vi "动力和环境监控系统状态详情.vi"() -> ()   [LabVIEW 2016, in "环境动力监测库.lvlib"]
uses:
  <vilib>/Utility/miscctls.llb/LVRowAndColumnTypeDef.ctl
  <vilib>/ptbypt/NI_PtbyPt.lvlib
panel:
  in  "监测设备更新":bool
  in  "设备列表":i32(listbox)
  in  "add":bool
  out "设备当前时间:":timestamp format="%<%Y/%m/%d %H:%M:%S>T"
  out "当前传感器数量:":i32
  in  "设备":T1(ring)
  # "系统当前状态"
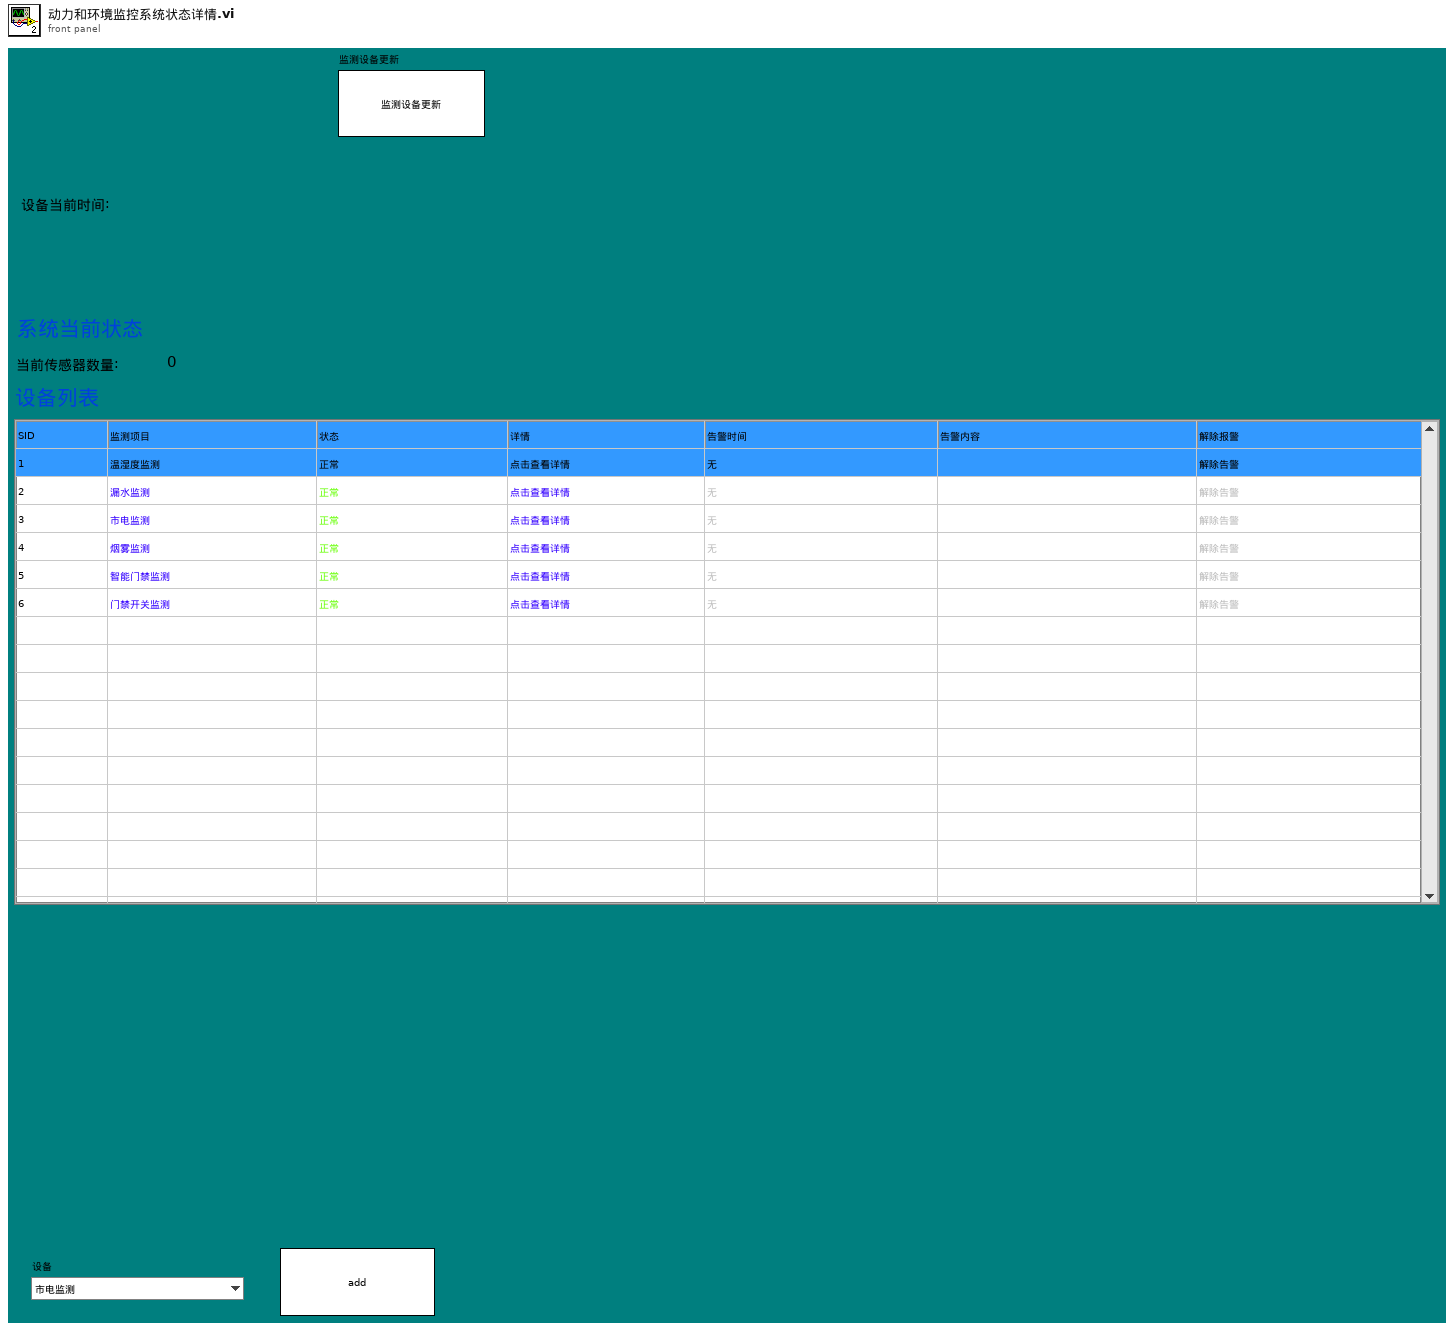
[diagram p1: front panel]
types:
  T1 = enum16{"市电监测", "UPS监测", "用水量监测", "空调监测", "烟雾监测", "温度湿度", "振动监测", "红外入侵监测", "漏水监测", "门禁开关监测", "视频监测"}
  T2 = cluster{"市电监测":bool, "用水量监测":bool, "烟雾监测":bool, "温度湿度":bool, "振动监测":bool, "红外入侵监测":bool, "漏水监测":bool, "门禁开关监测":bool, "门禁开关监测2":bool, "视频监测":bool, "UPS监测":bool, "空调监测":bool, "冰箱监测":bool, "排气扇监测":bool, "蓄电池监测":bool, "蓄电池监测2":bool, "GPS监测":bool, "北斗监测":bool, "气象监测":bool, "智能门禁监测":bool, "废液监测":bool, "废液监测2":bool, "灭火装置监测":bool}
  T3 = cluster{"漏水监测输出":cluster{"漏水监测告警":bool, "告警内容":string}, "门禁监测输出":cluster{"门禁监测告警":bool, "告警内容":string}, "门禁监测输出2":cluster{"门禁监测告警":bool, "告警内容":string}, "温湿度监测输出":cluster{"温湿度监测告警":bool, "告警内容":string}, "烟雾监测输出":cluster{"烟雾监测告警":bool, "告警内容":string}, "空调监测输出":cluster{"空调监测告警":bool, "告警内容":string}, "自动重合闸输出":cluster{"自动重合闸告警":bool, "告警内容":string}, "红外入侵输出":cluster{"红外入侵告警":bool, "告警内容":string}, "振动输出":cluster{"振动告警":bool, "告警内容":string}, "UPS输出":cluster{"UPS告警":bool, "告警内容":string}, "蓄电池输出":cluster{"蓄电池告警":bool, "告警内容":string}, "蓄电池输出2":cluster{"蓄电池告警":bool, "告警内容":string}, "GPS输出":cluster{"定位告警":bool, "告警内容":string}, "北斗输出":cluster{"定位告警":bool, "告警内容":string}, "气象输出":cluster{"气象告警":bool, "告警内容":string}, "废液输出":cluster{"废液告警":bool, "告警内容":string}, "废液输出2":cluster{"废液告警":bool, "告警内容":string}, "灭火装置输出":cluster{"灭火装置告警":bool, "告警内容":string}}
  T4 = cluster{"温湿度":cluster{"状态":bool, "温度:":sgl, "湿度:":sgl, "详情  ":bool}, "空调":cluster{"状态":bool, "机柜温度:":sgl, "压缩机:":enum16{"停止", "运行"}, "电加热:":enum16{"停止", "运行"}, "详情  ":bool}, "排气扇":cluster{"排气扇":bool, "详情  ":bool}, "冰箱":cluster{"冰箱":bool, "详情  ":bool}}
  T5 = cluster{"市电":cluster{"状态":bool, "电压:":u16, "电流：":dbl, "详情  ":bool}, "UPS":cluster{"状态":bool, "输入电压:":sgl, "输出电压:":sgl, "电池电量:":u8, "电量":u16, "详情  ":bool}, "蓄电池12V":cluster{"状态":bool, "电压:":sgl, "电流:":sgl, "电池电量:":u8, "电量":u16, "详情  ":bool, "充电":bool, "负载":bool}, "蓄电池24V":cluster{"状态":bool, "电压:":sgl, "电流:":sgl, "电池电量:":u8, "电量":u16, "详情  ":bool, "充电":bool, "负载":bool}}
  T6 = cluster{"传感器":cluster{"红外监测":cluster{"红外监测":bool, "红外入侵监测":bool}, "振动监测":cluster{"振动监测":bool, "振动监测 2":bool}, "烟雾监测":cluster{"烟雾监测":bool, "烟雾监测 2":bool}, "门禁监测":cluster{"门禁监测":bool, "门禁开关监测":bool}, "门禁2监测":cluster{"门禁监测2":bool, "门禁开关监测2":bool}, "水浸监测":cluster{"水浸监测":bool, "漏水详情":bool}, "废液监测":cluster{"废液监测":bool, "废液详情":bool}, "废液监测2":cluster{"废液监测2":bool, "废液2详情":bool}, "灭火装置":cluster{"灭火装置":bool, "灭火装置详情":bool}}, "气象仪":cluster{"气温: ":sgl, "气压: ":sgl, "风速:":sgl, "风向:":sgl, "气象仪经度: ":sgl, "气象仪纬度: ":sgl, "详情  ":bool}}
  T7 = cluster{"AD0":dbl, "AD1":dbl, "AD2":dbl, "AD3":dbl, "AD4":dbl, "AD5":dbl, "AD6":dbl, "AD7":dbl}
  T8 = cluster{"X0":dbl, "X1":dbl, "Y0":dbl, "Y1":dbl}[]
  T9 = enum32{"Invalid", "Standard", "Closed", "Hidden", "Minimized", "Maximized"}
  T10 = typedef "LVRowAndColumnTypeDef.ctl" = cluster{"Row":i32, "Column":i32}
  T11 = typedef "LVPoint32TypeDef.ctl" = cluster{"Horizontal":i32, "Vertical":i32}
  T12 = enum32{"Bad", "Idle", "Run top level", "Running"}
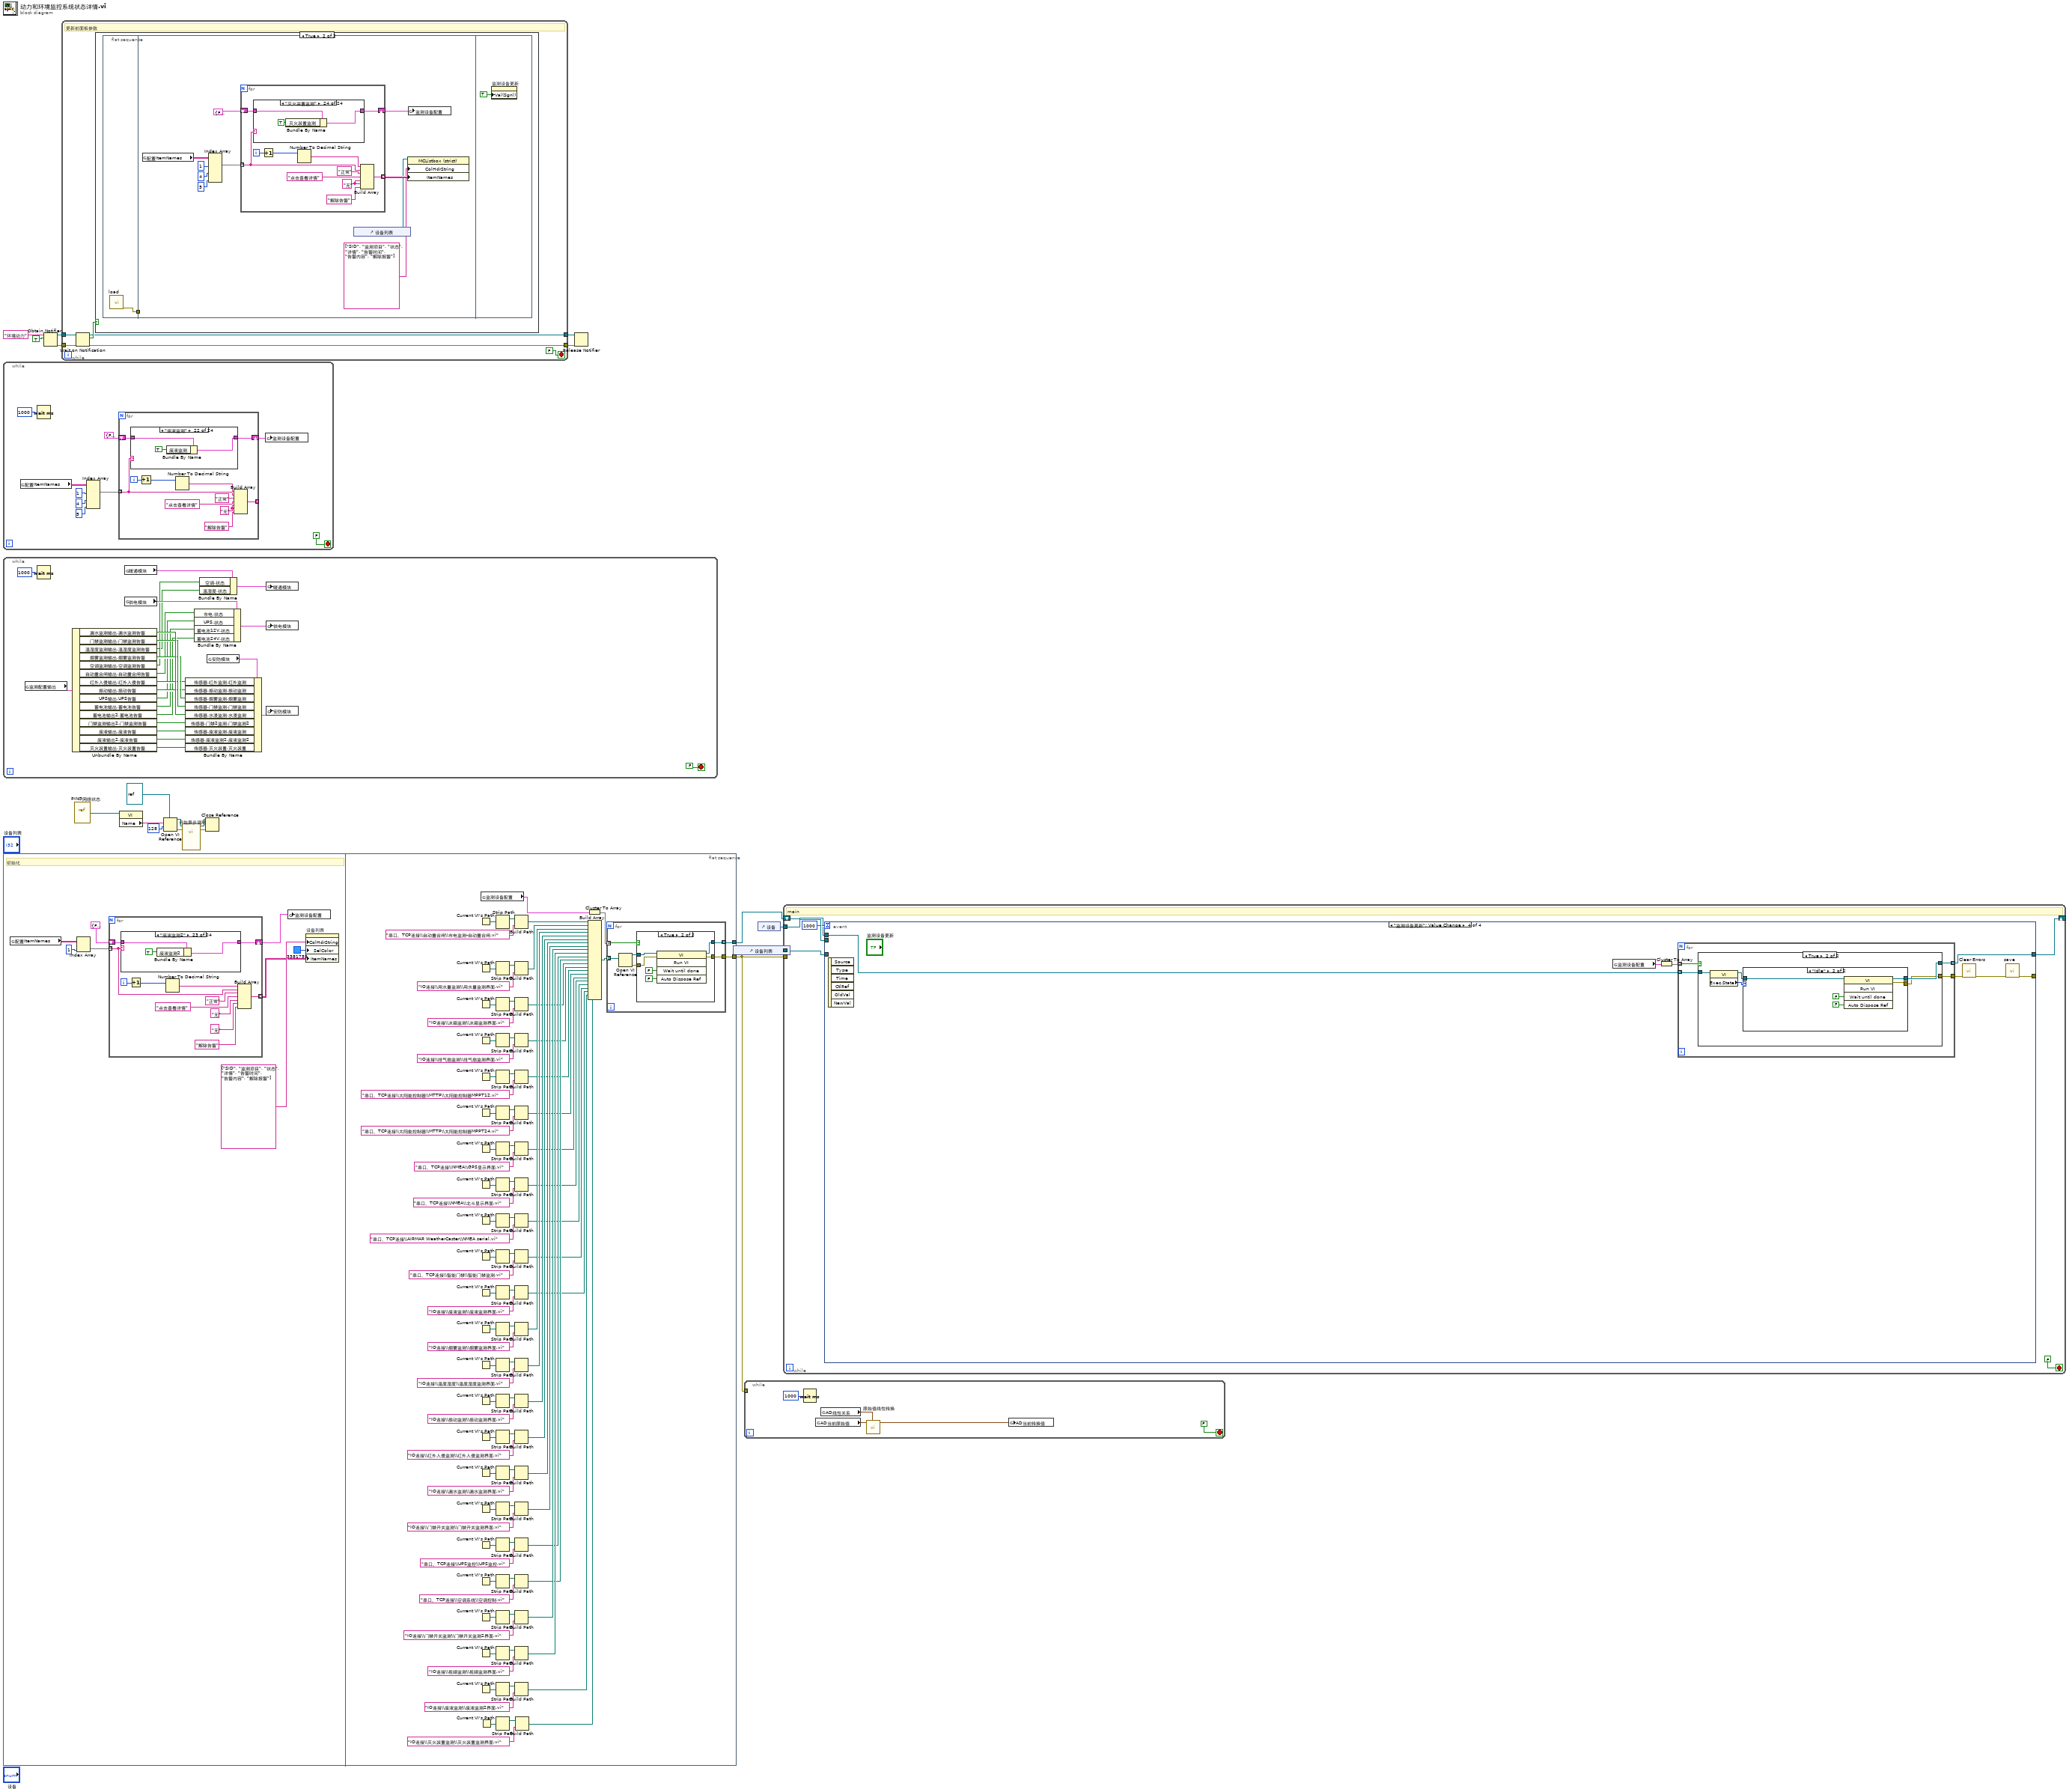
[diagram p0: block diagram]
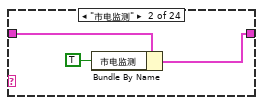
[diagram p3: hidden frame]
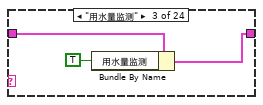
[diagram p4: hidden frame]
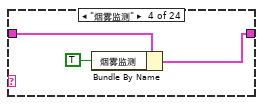
[diagram p5: hidden frame]
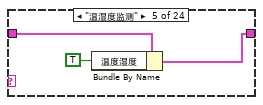
[diagram p6: hidden frame]
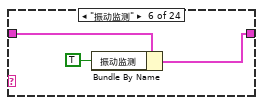
[diagram p7: hidden frame]
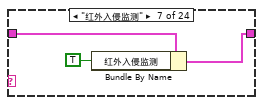
[diagram p8: hidden frame]
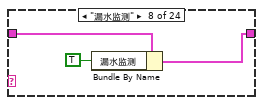
[diagram p9: hidden frame]
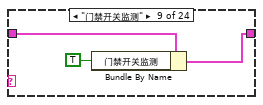
[diagram p10: hidden frame]
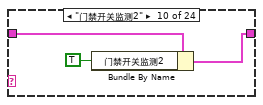
[diagram p11: hidden frame]
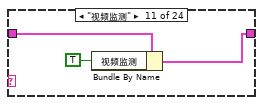
[diagram p12: hidden frame]
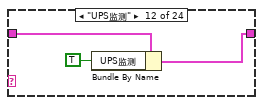
[diagram p13: hidden frame]
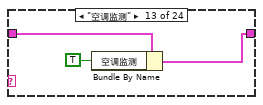
[diagram p14: hidden frame]
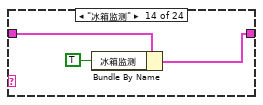
[diagram p15: hidden frame]
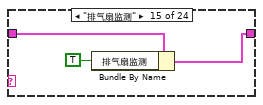
[diagram p16: hidden frame]
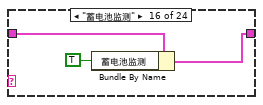
[diagram p17: hidden frame]
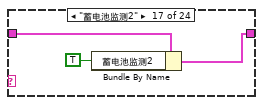
[diagram p18: hidden frame]
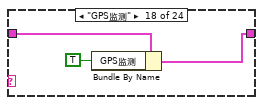
[diagram p19: hidden frame]
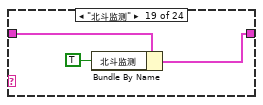
[diagram p20: hidden frame]
diagram:
  n1 = while {
    stop <- FALSE stop-if-true
    n2 = global read "断电保存全局变量.vi" "配置ItemNames"() -> (w22:string[][])
    n3 = Wait (ms)(milliseconds to wait=u32 1000 ("等待时间（毫秒）")) -> ()  [unwired: 1 out]
    n4 = Index Array(array=w22, index (col) #1=1 ("禁用的索引 (列)"), index (col) #2=4 ("索引 (列)"), index (col) #3=5 ("索引 (列)")) -> (element #1=w20:string[])  [unwired: 3 in, 2 out]
    n5 = for {
      tunnel: w20 -> [w29] mode=indexing
      tunnel: [w33] -> _ mode=indexing
      shift-right: [w28] -> w23
      shift-left: T2 {"市电监测"=FALSE, "用水量监测"=FALSE, "烟雾监测"=FALSE, "温度湿度"=FALSE, "振动监测"=FALSE, "红外入侵监测"=FALSE, "漏水监测"=FALSE, "门禁开关监测"=FALSE, "门禁开关监测2"=FALSE, "视频监测"=FALSE, "UPS监测"=FALSE, "空调监测"=FALSE, "冰箱监测"=FALSE, "排气扇监测"=FALSE, "蓄电池监测"=FALSE, "蓄电池监测2"=FALSE, "GPS监测"=FALSE, "北斗监测"=FALSE, "气象监测"=FALSE, "智能门禁监测"=FALSE, "废液监测"=FALSE, "废液监测2"=FALSE, "灭火装置监测"=FALSE} ("监测设备配置") -> [w30]
      i -> [w38]
      w31 = "无" ("元素")
      n6 = case shown="\"废液监测\"" w29 {
        tunnel: w30 -> [w39 w42 w44 w47 w50 w53 w56 w59 w62 w65 w68 w71 w74 w77 w80 w83 w86 w89 w92 w95 w98 w101 w104 w107]
        tunnel: [w39 w40 w43 w46 w49 w52 w55 w58 w61 w64 w67 w70 w73 w76 w79 w82 w85 w88 w91 w94 w97 w100 w103 w106] -> w28
        frame "假", Default {
        }
        frame "市电监测" {
          n7 = Bundle By Name(cluster=w42, "市电监测"=TRUE) -> (w40:T2)
        }
        frame "用水量监测" {
          n8 = Bundle By Name(cluster=w44, "用水量监测"=TRUE ("市电监测")) -> (w43:T2)
        }
        frame "烟雾监测" {
          n9 = Bundle By Name(cluster=w47, "烟雾监测"=TRUE ("市电监测")) -> (w46:T2)
        }
        frame "温湿度监测" {
          n10 = Bundle By Name(cluster=w50, "温度湿度"=TRUE ("市电监测")) -> (w49:T2)
        }
        frame "振动监测" {
          n11 = Bundle By Name(cluster=w53, "振动监测"=TRUE ("市电监测")) -> (w52:T2)
        }
        frame "红外入侵监测" {
          n12 = Bundle By Name(cluster=w56, "红外入侵监测"=TRUE ("市电监测")) -> (w55:T2)
        }
        frame "漏水监测" {
          n13 = Bundle By Name(cluster=w59, "漏水监测"=TRUE ("市电监测")) -> (w58:T2)
        }
        frame "门禁开关监测" {
          n14 = Bundle By Name(cluster=w62, "门禁开关监测"=TRUE ("市电监测")) -> (w61:T2)
        }
        frame "门禁开关监测2" {
          n15 = Bundle By Name(cluster=w65, "门禁开关监测2"=TRUE ("市电监测")) -> (w64:T2)
        }
        frame "视频监测" {
          n16 = Bundle By Name(cluster=w68, "视频监测"=TRUE ("市电监测")) -> (w67:T2)
        }
        frame "UPS监测" {
          n17 = Bundle By Name(cluster=w71, "UPS监测"=TRUE ("市电监测")) -> (w70:T2)
        }
        frame "空调监测" {
          n18 = Bundle By Name(cluster=w74, "空调监测"=TRUE ("市电监测")) -> (w73:T2)
        }
        frame "冰箱监测" {
          n19 = Bundle By Name(cluster=w77, "冰箱监测"=TRUE ("市电监测")) -> (w76:T2)
        }
        frame "排气扇监测" {
          n20 = Bundle By Name(cluster=w80, "排气扇监测"=TRUE ("市电监测")) -> (w79:T2)
        }
        frame "蓄电池监测" {
          n21 = Bundle By Name(cluster=w83, "蓄电池监测"=TRUE ("市电监测")) -> (w82:T2)
        }
        frame "蓄电池监测2" {
          n22 = Bundle By Name(cluster=w86, "蓄电池监测2"=TRUE ("市电监测")) -> (w85:T2)
        }
        frame "GPS监测" {
          n23 = Bundle By Name(cluster=w89, "GPS监测"=TRUE ("市电监测")) -> (w88:T2)
        }
        frame "北斗监测" {
          n24 = Bundle By Name(cluster=w92, "北斗监测"=TRUE ("市电监测")) -> (w91:T2)
        }
        frame "气象监测" {
          n25 = Bundle By Name(cluster=w95, "气象监测"=TRUE ("市电监测")) -> (w94:T2)
        }
        frame "智能门禁监测" {
          n26 = Bundle By Name(cluster=w98, "智能门禁监测"=TRUE ("市电监测")) -> (w97:T2)
        }
        frame "废液监测" {
          n27 = Bundle By Name(cluster=w101, "废液监测"=TRUE ("市电监测")) -> (w100:T2)
        }
        frame "废液监测2" {
          n28 = Bundle By Name(cluster=w104, "废液监测2"=TRUE ("市电监测")) -> (w103:T2)
        }
        frame "灭火装置监测" {
          n29 = Bundle By Name(cluster=w107, "灭火装置监测"=TRUE ("市电监测")) -> (w106:T2)
        }
      }
      n30 = Increment(x=w38) -> (x+1=w37:i32)
      n31 = Number To Decimal String(number=w37) -> (decimal integer string=w36:string)  [unwired: 1 in]
      n32 = Build Array(w36, w29, "正常" ("元素"), "点击查看详情" ("元素"), w31, w31, "解除告警" ("元素")) -> (w33:string[])
    }
    n33 = global write "断电保存全局变量.vi" "监测设备配置"(w23) -> ()
  }
  n34 = while {
    stop <- FALSE stop-if-true
    n35 = global read "内部交互全局变量.vi" "监测配置输出"() -> (w113:T3)
    n36 = Wait (ms)(milliseconds to wait=u32 1000 ("等待时间（毫秒）")) -> ()  [unwired: 1 out]
    n37 = Unbundle By Name(w113) -> ("漏水监测输出.漏水监测告警"=w128:bool, "门禁监测输出.门禁监测告警"=w127:bool, "温湿度监测输出.温湿度监测告警"=w115:bool, "烟雾监测输出.烟雾监测告警"=w126:bool, "空调监测输出.空调监测告警"=w116:bool, "自动重合闸输出.自动重合闸告警"=w121:bool, "红外入侵输出.红外入侵告警"=w125:bool, "振动输出.振动告警"=w124:bool, "UPS输出.UPS告警"=w120:bool, "蓄电池输出.蓄电池告警"=w119:bool, "蓄电池输出2.蓄电池告警"=w114:bool, "门禁监测输出2.门禁监测告警"=w112:bool, "废液输出.废液告警"=w111:bool, "废液输出2.废液告警"=w110:bool, "灭火装置输出.灭火装置告警"=w109:bool)
    n38 = global read "内部交互全局变量.vi" "暖通模块"() -> (w118:T4)
    n39 = global read "内部交互全局变量.vi" "供电模块"() -> (w122:T5)
    n40 = Bundle By Name(cluster=w122, "市电.状态"=w121, "UPS.状态"=w120, "蓄电池12V.状态"=w119, "蓄电池24V.状态"=w114) -> (w123:T5)
    n41 = Bundle By Name(cluster=w118, "空调.状态"=w116, "温湿度.状态"=w115) -> (w117:T4)
    n42 = global read "内部交互全局变量.vi" "安防模块"() -> (w130:T6)
    n43 = Bundle By Name(cluster=w130, "传感器.红外监测.红外监测"=w125, "传感器.振动监测.振动监测"=w124, "传感器.烟雾监测.烟雾监测"=w126, "传感器.门禁监测.门禁监测"=w127, "传感器.水浸监测.水浸监测"=w128, "传感器.门禁2监测.门禁监测2"=w112, "传感器.废液监测.废液监测"=w111, "传感器.废液监测2.废液监测2"=w110, "传感器.灭火装置.灭火装置"=w109) -> (w129:T6)
    n44 = global write "内部交互全局变量.vi" "暖通模块"(w117) -> ()
    n45 = global write "内部交互全局变量.vi" "供电模块"(w123) -> ()
    n46 = global write "内部交互全局变量.vi" "安防模块"(w129) -> ()
  }
  n47 = flat-sequence {
    tunnel: [w317] -> w12
    tunnel: [w227] -> w1
    frame #0 {
      # "初始化"
      n48 = global read "断电保存全局变量.vi" "配置ItemNames"() -> (w138:string[][])
      n49 = Index Array(array=w138, index (col)=1 ("禁用的索引 (列)")) -> (element=w136:string[])  [unwired: 1 in]
      n50 = for {
        tunnel: w136 -> [w143] mode=indexing
        tunnel: [w147] -> w135 mode=indexing
        shift-right: [w141] -> w133
        shift-left: T2 {"市电监测"=FALSE, "用水量监测"=FALSE, "烟雾监测"=FALSE, "温度湿度"=FALSE, "振动监测"=FALSE, "红外入侵监测"=FALSE, "漏水监测"=FALSE, "门禁开关监测"=FALSE, "门禁开关监测2"=FALSE, "视频监测"=FALSE, "UPS监测"=FALSE, "空调监测"=FALSE, "冰箱监测"=FALSE, "排气扇监测"=FALSE, "蓄电池监测"=FALSE, "蓄电池监测2"=FALSE, "GPS监测"=FALSE, "北斗监测"=FALSE, "气象监测"=FALSE, "智能门禁监测"=FALSE, "废液监测"=FALSE, "废液监测2"=FALSE, "灭火装置监测"=FALSE} ("监测设备配置") -> [w142]
        i -> [w152]
        n51 = case shown="\"废液监测2\"" w143 {
          tunnel: w142 -> [w153 w156 w158 w161 w164 w167 w170 w173 w176 w179 w182 w185 w188 w191 w194 w197 w200 w203 w206 w209 w212 w215 w218 w221]
          tunnel: [w153 w154 w157 w160 w163 w166 w169 w172 w175 w178 w181 w184 w187 w190 w193 w196 w199 w202 w205 w208 w211 w214 w217 w220] -> w141
          frame "假", Default {
          }
          frame "市电监测" {
            n52 = Bundle By Name(cluster=w156, "市电监测"=TRUE) -> (w154:T2)
          }
          frame "用水量监测" {
            n53 = Bundle By Name(cluster=w158, "用水量监测"=TRUE ("市电监测")) -> (w157:T2)
          }
          frame "烟雾监测" {
            n54 = Bundle By Name(cluster=w161, "烟雾监测"=TRUE ("市电监测")) -> (w160:T2)
          }
          frame "温湿度监测" {
            n55 = Bundle By Name(cluster=w164, "温度湿度"=TRUE ("市电监测")) -> (w163:T2)
          }
          frame "振动监测" {
            n56 = Bundle By Name(cluster=w167, "振动监测"=TRUE ("市电监测")) -> (w166:T2)
          }
          frame "红外入侵监测" {
            n57 = Bundle By Name(cluster=w170, "红外入侵监测"=TRUE ("市电监测")) -> (w169:T2)
          }
          frame "漏水监测" {
            n58 = Bundle By Name(cluster=w173, "漏水监测"=TRUE ("市电监测")) -> (w172:T2)
          }
          frame "门禁开关监测" {
            n59 = Bundle By Name(cluster=w176, "门禁开关监测"=TRUE ("市电监测")) -> (w175:T2)
          }
          frame "门禁开关监测2" {
            n60 = Bundle By Name(cluster=w179, "门禁开关监测2"=TRUE ("市电监测")) -> (w178:T2)
          }
          frame "视频监测" {
            n61 = Bundle By Name(cluster=w182, "视频监测"=TRUE ("市电监测")) -> (w181:T2)
          }
          frame "UPS监测" {
            n62 = Bundle By Name(cluster=w185, "UPS监测"=TRUE ("市电监测")) -> (w184:T2)
          }
          frame "空调监测" {
            n63 = Bundle By Name(cluster=w188, "空调监测"=TRUE ("市电监测")) -> (w187:T2)
          }
          frame "冰箱监测" {
            n64 = Bundle By Name(cluster=w191, "冰箱监测"=TRUE ("市电监测")) -> (w190:T2)
          }
          frame "排气扇监测" {
            n65 = Bundle By Name(cluster=w194, "排气扇监测"=TRUE ("市电监测")) -> (w193:T2)
          }
          frame "蓄电池监测" {
            n66 = Bundle By Name(cluster=w197, "蓄电池监测"=TRUE ("市电监测")) -> (w196:T2)
          }
          frame "蓄电池监测2" {
            n67 = Bundle By Name(cluster=w200, "蓄电池监测2"=TRUE ("市电监测")) -> (w199:T2)
          }
          frame "GPS监测" {
            n68 = Bundle By Name(cluster=w203, "GPS监测"=TRUE ("市电监测")) -> (w202:T2)
          }
          frame "北斗监测" {
            n69 = Bundle By Name(cluster=w206, "北斗监测"=TRUE ("市电监测")) -> (w205:T2)
          }
          frame "气象监测" {
            n70 = Bundle By Name(cluster=w209, "气象监测"=TRUE ("市电监测")) -> (w208:T2)
          }
          frame "智能门禁监测" {
            n71 = Bundle By Name(cluster=w212, "智能门禁监测"=TRUE ("市电监测")) -> (w211:T2)
          }
          frame "废液监测" {
            n72 = Bundle By Name(cluster=w215, "废液监测"=TRUE ("市电监测")) -> (w214:T2)
          }
          frame "废液监测2" {
            n73 = Bundle By Name(cluster=w218, "废液监测2"=TRUE ("市电监测")) -> (w217:T2)
          }
          frame "灭火装置监测" {
            n74 = Bundle By Name(cluster=w221, "灭火装置监测"=TRUE ("市电监测")) -> (w220:T2)
          }
        }
        n75 = Increment(x=w152) -> (x+1=w151:i32)
        n76 = Number To Decimal String(number=w151) -> (decimal integer string=w150:string)  [unwired: 1 in]
        n77 = Build Array(w150, w143, "正常" ("元素"), "点击查看详情" ("元素"), "无" ("元素"), "无" ("元素"), "解除告警" ("元素")) -> (w147:string[])
      }
      n78 = global write "断电保存全局变量.vi" "监测设备配置"(w133) -> ()
      n79 = property on="设备列表" class="MCListbox (strict)"("ColHdrString"=string[] ["SID", "监测项目", "状态", "详情", "告警时间", "告警内容", "解除报警"] ("列首字符串[]"), "SelColor"=u32 3381759, "ItemNames"=w135) -> ()  [unwired: 2 in, 2 out]
    }
    frame #1 {
      n80 = Current VI's Path() -> (path=w315:path)
      n81 = Current VI's Path() -> (path=w309:path)
      n82 = Current VI's Path() -> (path=w264:path)
      n83 = Current VI's Path() -> (path=w265:path)
      n84 = Current VI's Path() -> (path=w259:path)
      n85 = Current VI's Path() -> (path=w254:path)
      n86 = Current VI's Path() -> (path=w251:path)
      n87 = Current VI's Path() -> (path=w245:path)
      n88 = Current VI's Path() -> (path=w243:path)
      n89 = Current VI's Path() -> (path=w237:path)
      n90 = Current VI's Path() -> (path=w235:path)
      n91 = Current VI's Path() -> (path=w307:path)
      n92 = Current VI's Path() -> (path=w301:path)
      n93 = Current VI's Path() -> (path=w299:path)
      n94 = Current VI's Path() -> (path=w293:path)
      n95 = Current VI's Path() -> (path=w289:path)
      n96 = Current VI's Path() -> (path=w287:path)
      n97 = Current VI's Path() -> (path=w275:path)
      n98 = Current VI's Path() -> (path=w269:path)
      n99 = Current VI's Path() -> (path=w281:path)
      n100 = Current VI's Path() -> (path=w279:path)
      n101 = Current VI's Path() -> (path=w230:path)
      n102 = Current VI's Path() -> (path=w226:path)
      n103 = global read "断电保存全局变量.vi" "监测设备配置"() -> (w316:T2)
      n104 = Strip Path(path=w315) -> (stripped path=w314:path)  [unwired: 1 out]
      n105 = Strip Path(path=w309) -> (stripped path=w310:path)  [unwired: 1 out]
      n106 = Strip Path(path=w264) -> (stripped path=w263:path)  [unwired: 1 out]
      n107 = Strip Path(path=w265) -> (stripped path=w266:path)  [unwired: 1 out]
      n108 = Strip Path(path=w259) -> (stripped path=w258:path)  [unwired: 1 out]
      n109 = Strip Path(path=w254) -> (stripped path=w255:path)  [unwired: 1 out]
      n110 = Strip Path(path=w251) -> (stripped path=w250:path)  [unwired: 1 out]
      n111 = Strip Path(path=w245) -> (stripped path=w246:path)  [unwired: 1 out]
      n112 = Strip Path(path=w243) -> (stripped path=w242:path)  [unwired: 1 out]
      n113 = Strip Path(path=w237) -> (stripped path=w238:path)  [unwired: 1 out]
      n114 = Strip Path(path=w235) -> (stripped path=w234:path)  [unwired: 1 out]
      n115 = Strip Path(path=w307) -> (stripped path=w306:path)  [unwired: 1 out]
      n116 = Strip Path(path=w301) -> (stripped path=w302:path)  [unwired: 1 out]
      n117 = Strip Path(path=w299) -> (stripped path=w298:path)  [unwired: 1 out]
      n118 = Strip Path(path=w293) -> (stripped path=w294:path)  [unwired: 1 out]
      n119 = Strip Path(path=w289) -> (stripped path=w290:path)  [unwired: 1 out]
      n120 = Strip Path(path=w287) -> (stripped path=w286:path)  [unwired: 1 out]
      n121 = Strip Path(path=w275) -> (stripped path=w274:path)  [unwired: 1 out]
      n122 = Strip Path(path=w269) -> (stripped path=w270:path)  [unwired: 1 out]
      n123 = Strip Path(path=w281) -> (stripped path=w282:path)  [unwired: 1 out]
      n124 = Strip Path(path=w279) -> (stripped path=w278:path)  [unwired: 1 out]
      n125 = Strip Path(path=w230) -> (stripped path=w231:path)  [unwired: 1 out]
      n126 = Strip Path(path=w226) -> (stripped path=w225:path)  [unwired: 1 out]
      n127 = Build Path(base path=w314, name or relative path="串口、TCP连接\\自动重合闸\\市电监测-自动重合闸.vi" ("名称或相对路径")) -> (appended path=w312:path)
      n128 = Build Path(base path=w310, name or relative path="IO连接\\用水量监测\\用水量监测界面.vi" ("名称或相对路径")) -> (appended path=w308:path)
      n129 = Build Path(base path=w263, name or relative path="IO连接\\冰箱监测\\冰箱监测界面.vi" ("名称或相对路径")) -> (appended path=w261:path)
      n130 = Build Path(base path=w266, name or relative path="IO连接\\排气扇监测\\排气扇监测界面.vi" ("名称或相对路径")) -> (appended path=w260:path)
      n131 = Build Path(base path=w258, name or relative path="串口、TCP连接\\太阳能控制器\\MTTP\\太阳能控制器MPPT12.vi" ("名称或相对路径")) -> (appended path=w253:path)
      n132 = Build Path(base path=w255, name or relative path="串口、TCP连接\\太阳能控制器\\MTTP\\太阳能控制器MPPT24.vi" ("名称或相对路径")) -> (appended path=w252:path)
      n133 = Build Path(base path=w250, name or relative path="串口、TCP连接\\NMEA\\GPS显示界面.vi" ("名称或相对路径")) -> (appended path=w248:path)
      n134 = Build Path(base path=w246, name or relative path="串口、TCP连接\\NMEA\\北斗显示界面.vi" ("名称或相对路径")) -> (appended path=w244:path)
      n135 = Build Path(base path=w242, name or relative path="串口、TCP连接\\AIRMAR WeatherCaster\\NMEA serial.vi" ("名称或相对路径")) -> (appended path=w240:path)
      n136 = Build Path(base path=w238, name or relative path="串口、TCP连接\\智能门禁\\智能门禁监测.vi" ("名称或相对路径")) -> (appended path=w236:path)
      n137 = Build Path(base path=w234, name or relative path="IO连接\\废液监测\\废液监测界面.vi" ("名称或相对路径")) -> (appended path=w229:path)
      n138 = Build Path(base path=w306, name or relative path="IO连接\\烟雾监测\\烟雾监测界面.vi" ("名称或相对路径")) -> (appended path=w304:path)
      n139 = Build Path(base path=w302, name or relative path="IO连接\\温度湿度\\温度湿度监测界面.vi" ("名称或相对路径")) -> (appended path=w300:path)
      n140 = Build Path(base path=w298, name or relative path="IO连接\\振动监测\\振动监测界面.vi" ("名称或相对路径")) -> (appended path=w296:path)
      n141 = Build Path(base path=w294, name or relative path="IO连接\\红外入侵监测\\红外入侵监测界面.vi" ("名称或相对路径")) -> (appended path=w292:path)
      n142 = Build Path(base path=w290, name or relative path="IO连接\\漏水监测\\漏水监测界面.vi" ("名称或相对路径")) -> (appended path=w288:path)
      n143 = Build Path(base path=w286, name or relative path="IO连接\\门禁开关监测\\门禁开关监测界面.vi" ("名称或相对路径")) -> (appended path=w284:path)
      n144 = Build Path(base path=w274, name or relative path="串口、TCP连接\\UPS监控\\UPS监控.vi" ("名称或相对路径")) -> (appended path=w272:path)
      n145 = Build Path(base path=w270, name or relative path="串口、TCP连接\\空调系统\\空调控制.vi" ("名称或相对路径")) -> (appended path=w268:path)
      n146 = Build Path(base path=w282, name or relative path="IO连接\\门禁开关监测\\门禁开关监测2界面.vi" ("名称或相对路径")) -> (appended path=w280:path)
      n147 = Build Path(base path=w278, name or relative path="IO连接\\视频监测\\视频监测界面.vi" ("名称或相对路径")) -> (appended path=w276:path)
      n148 = Build Path(base path=w231, name or relative path="IO连接\\废液监测\\废液监测2界面.vi" ("名称或相对路径")) -> (appended path=w228:path)
      n149 = Build Path(base path=w225, name or relative path="IO连接\\灭火装置监测\\灭火装置监测界面.vi" ("名称或相对路径")) -> (appended path=w223:path)
      n150 = Cluster To Array(cluster=w316) -> (array=w319:bool[])
      n151 = Build Array(w312, w308, w304, w300, w296, w292, w288, w284, w280, w276, w272, w268, w261, w260, w253, w252, w248, w244, w240, w236, w229, w228, w223) -> (w318:path[])
      n152 = for {
        tunnel: w318 -> [w322] mode=indexing
        tunnel: [w321] -> w317 mode=indexing
        tunnel: w319 -> [w325] mode=indexing
        tunnel: [w320] -> w227
        n153 = Open VI Reference(vi path=w322) -> (vi reference=w324:refnum<vi>, error out=w323:errorcluster)  [unwired: 5 in]
        n154 = case shown="True" w325 {
          tunnel: w324 -> [w326 w330]
          tunnel: [w326 w329] -> w321
          tunnel: [_ w328] -> w320
          tunnel: w323 -> [_ w327]
          frame False {
          }
          frame True {
            n155 = invoke class="VI" method="Run VI"(reference=w330, error in=w327, "Wait until done"=FALSE ("结束前等待"), "Auto Dispose Ref"=FALSE ("自动销毁引用")) -> (reference out=w329:refnum<vi>, error out=w328:errorcluster)  [unwired: 1 in, 3 out]
          }
        }
      }
    }
  }
  n156 = Obtain Notifier(name (unnamed)="环境动力" ("名称（未命名）"), notification data type=TRUE) -> (notifier out=w3:refnum<notifier>, error out=w2:errorcluster)  [unwired: 2 in, 1 out]
  n157 = while {
    tunnel: w3 -> [w338]
    tunnel: w2 -> [w337]
    tunnel: [w334] -> w14
    tunnel: [w333] -> w13
    stop <- FALSE stop-if-true
    # "更新前面板参数"
    n158 = Wait on Notification(notifier=w338, error in (no error)=w337) -> (notifier out=w334:refnum<notifier>, notification=w336:bool, error out=w333:errorcluster)  [unwired: 2 in, 1 out]
    n159 = case shown="True" w336 {
      frame False {
      }
      frame True {
        n160 = flat-sequence {
          tunnel: [w340] -> w339
          tunnel: w339 -> [_]
          frame #0 {
            n161 = call "load.vi"() -> ("error out"=w340:errorcluster)  [unwired: 11 in]
          }
          frame #1 {
            n162 = global read "断电保存全局变量.vi" "配置ItemNames"() -> (w345:string[][])
            n163 = Index Array(array=w345, index (col) #1=1 ("禁用的索引 (列)"), index (col) #2=4 ("索引 (列)"), index (col) #3=5 ("索引 (列)")) -> (element #1=w347:string[])  [unwired: 3 in, 2 out]
            n164 = for {
              tunnel: w347 -> [w352] mode=indexing
              tunnel: [w356] -> w350 mode=indexing
              shift-right: [w351] -> w342
              shift-left: T2 {"市电监测"=FALSE, "用水量监测"=FALSE, "烟雾监测"=FALSE, "温度湿度"=FALSE, "振动监测"=FALSE, "红外入侵监测"=FALSE, "漏水监测"=FALSE, "门禁开关监测"=FALSE, "门禁开关监测2"=FALSE, "视频监测"=FALSE, "UPS监测"=FALSE, "空调监测"=FALSE, "冰箱监测"=FALSE, "排气扇监测"=FALSE, "蓄电池监测"=FALSE, "蓄电池监测2"=FALSE, "GPS监测"=FALSE, "北斗监测"=FALSE, "气象监测"=FALSE, "智能门禁监测"=FALSE, "废液监测"=FALSE, "废液监测2"=FALSE, "灭火装置监测"=FALSE} ("监测设备配置") -> [w353]
              i -> [w361]
              w354 = "无" ("元素")
              n165 = case shown="\"灭火装置监测\"" w352 {
                tunnel: w353 -> [w362 w365 w367 w370 w373 w376 w379 w382 w385 w388 w391 w394 w397 w400 w403 w406 w409 w412 w415 w418 w421 w424 w427 w430]
                tunnel: [w362 w363 w366 w369 w372 w375 w378 w381 w384 w387 w390 w393 w396 w399 w402 w405 w408 w411 w414 w417 w420 w423 w426 w429] -> w351
                frame "假", Default {
                }
                frame "市电监测" {
                  n166 = Bundle By Name(cluster=w365, "市电监测"=TRUE) -> (w363:T2)
                }
                frame "用水量监测" {
                  n167 = Bundle By Name(cluster=w367, "用水量监测"=TRUE ("市电监测")) -> (w366:T2)
                }
                frame "烟雾监测" {
                  n168 = Bundle By Name(cluster=w370, "烟雾监测"=TRUE ("市电监测")) -> (w369:T2)
                }
                frame "温湿度监测" {
                  n169 = Bundle By Name(cluster=w373, "温度湿度"=TRUE ("市电监测")) -> (w372:T2)
                }
                frame "振动监测" {
                  n170 = Bundle By Name(cluster=w376, "振动监测"=TRUE ("市电监测")) -> (w375:T2)
                }
                frame "红外入侵监测" {
                  n171 = Bundle By Name(cluster=w379, "红外入侵监测"=TRUE ("市电监测")) -> (w378:T2)
                }
                frame "漏水监测" {
                  n172 = Bundle By Name(cluster=w382, "漏水监测"=TRUE ("市电监测")) -> (w381:T2)
                }
                frame "门禁开关监测" {
                  n173 = Bundle By Name(cluster=w385, "门禁开关监测"=TRUE ("市电监测")) -> (w384:T2)
                }
                frame "门禁开关监测2" {
                  n174 = Bundle By Name(cluster=w388, "门禁开关监测2"=TRUE ("市电监测")) -> (w387:T2)
                }
                frame "视频监测" {
                  n175 = Bundle By Name(cluster=w391, "视频监测"=TRUE ("市电监测")) -> (w390:T2)
                }
                frame "UPS监测" {
                  n176 = Bundle By Name(cluster=w394, "UPS监测"=TRUE ("市电监测")) -> (w393:T2)
                }
                frame "空调监测" {
                  n177 = Bundle By Name(cluster=w397, "空调监测"=TRUE ("市电监测")) -> (w396:T2)
                }
                frame "冰箱监测" {
                  n178 = Bundle By Name(cluster=w400, "冰箱监测"=TRUE ("市电监测")) -> (w399:T2)
                }
                frame "排气扇监测" {
                  n179 = Bundle By Name(cluster=w403, "排气扇监测"=TRUE ("市电监测")) -> (w402:T2)
                }
                frame "蓄电池监测" {
                  n180 = Bundle By Name(cluster=w406, "蓄电池监测"=TRUE ("市电监测")) -> (w405:T2)
                }
                frame "蓄电池监测2" {
                  n181 = Bundle By Name(cluster=w409, "蓄电池监测2"=TRUE ("市电监测")) -> (w408:T2)
                }
                frame "GPS监测" {
                  n182 = Bundle By Name(cluster=w412, "GPS监测"=TRUE ("市电监测")) -> (w411:T2)
                }
                frame "北斗监测" {
                  n183 = Bundle By Name(cluster=w415, "北斗监测"=TRUE ("市电监测")) -> (w414:T2)
                }
                frame "气象监测" {
                  n184 = Bundle By Name(cluster=w418, "气象监测"=TRUE ("市电监测")) -> (w417:T2)
                }
                frame "智能门禁监测" {
                  n185 = Bundle By Name(cluster=w421, "智能门禁监测"=TRUE ("市电监测")) -> (w420:T2)
                }
                frame "废液监测" {
                  n186 = Bundle By Name(cluster=w424, "废液监测"=TRUE ("市电监测")) -> (w423:T2)
                }
                frame "废液监测2" {
                  n187 = Bundle By Name(cluster=w427, "废液监测2"=TRUE ("市电监测")) -> (w426:T2)
                }
                frame "灭火装置监测" {
                  n188 = Bundle By Name(cluster=w430, "灭火装置监测"=TRUE ("市电监测")) -> (w429:T2)
                }
              }
              n189 = Increment(x=w361) -> (x+1=w360:i32)
              n190 = Number To Decimal String(number=w360) -> (decimal integer string=w359:string)  [unwired: 1 in]
              n191 = Build Array(w359, w352, "正常" ("元素"), "点击查看详情" ("元素"), w354, w354, "解除告警" ("元素")) -> (w356:string[])
            }
            n192 = control-ref of="设备列表"() -> (w348:refnum<vi>)
            n193 = property class="MCListbox (strict)"(reference=w348, "ColHdrString"=string[] ["SID", "监测项目", "状态", "详情", "告警时间", "告警内容", "解除报警"] ("列首字符串[]"), "ItemNames"=w350) -> ()  [unwired: 1 in, 2 out]
            n194 = global write "断电保存全局变量.vi" "监测设备配置"(w342) -> ()
          }
          frame #2 {
            n195 = property on="监测设备更新" class="Bool (strict)"("Val(Sgnl)"=TRUE ("值(信号)")) -> ()  [unwired: 2 in, 2 out]
          }
        }
      }
    }
  }
  n196 = vi-ref "PING网络状态.vi"() -> (w4:refnum<vi>)
  n197 = property class="VI"(reference=w4) -> ("Name"=w11:string)  [unwired: 1 in, 2 out]
  n198 = Open VI Reference(type specifier VI Refnum (for type only)=refnum<vi> refnum, vi path=w11, options=128 ("选项")) -> (vi reference=w9:refnum<vi>, error out=w7:errorcluster)  [unwired: 3 in]
  n199 = call-by-ref "开始异步调用"(reference=w9, error in=w7) -> (reference out=w5:refnum<vi>, error out=w6:errorcluster)  [unwired: 12 in]
  n200 = Close Reference(reference=w5, error in (no error)=w6) -> ()  [unwired: 1 out]
  n201 = Release Notifier(notifier=w14, error in (no error)=w13) -> ()  [unwired: 1 in, 3 out]
  n202 = control-ref of="设备列表"() -> (w18:refnum<vi>)
  n203 = while {
    tunnel: w1 -> [_]
    stop <- FALSE stop-if-true
    n204 = Wait (ms)(milliseconds to wait=u32 1000 ("等待时间（毫秒）")) -> ()  [unwired: 1 out]
    n205 = global read "断电保存全局变量.vi" "AD当前原始值"() -> (w435:T7)
    n206 = global read "断电保存全局变量.vi" "AD线性关系"() -> (w433:T8)
    n207 = call "原始值线性转换.vi"("AD线性关系"=w433, "AD当前原始值"=w435) -> ("AD当前转换值"=w434:T7)  [unwired: 9 in]
    n208 = global write "断电保存全局变量.vi" "AD当前转换值"(w434) -> ()
  }
  n209 = control-ref of="设备"() -> (w17:refnum<vi>)
  n210 = while {
    tunnel: w18 -> [w442]
    tunnel: w17 -> [w441]
    tunnel: w1 -> [_]
    shift-right: [w438] -> _
    shift-left: w12 -> [w439]
    stop <- FALSE stop-if-true
    # "main"
    n211 = event shown="[3] \"监测设备更新\": Value Change" {
      selector: _ -> [_ _ _ _]
      dyn-events: _ -> [_ _ _ _]
      timeout: 1000 -> [_ _ _ _]
      tunnel: w442 -> [_ w618 w625 _]
      tunnel: w441 -> [_ w617 _ _]
      tunnel: w439 -> [w453 w592 w619 w772]
      tunnel: [w453 w592 w619 w771] -> w438
      tunnel: [_ _ _ w767] -> _
      event Timeout {
        n212 = event-data() -> ()  [unwired: 1 in, 3 out]
        n213 = Get Date/Time In Seconds() -> (seconds since 1Jan1904=→"设备当前时间:":timestamp)
        n214 = property on="设备列表" class="MCListbox (strict)"() -> (error out=w455:errorcluster, "ItemNames"=w464:string[][])  [unwired: 2 in, 1 out]
        n215 = global read "内部交互全局变量.vi" "监测配置输出"() -> (w444:T3)
        n216 = Array Size(array=w464) -> (size(s)=w470:i32[])
        n217 = Index Array(array=w464, index (col) #1=1 ("禁用的索引 (列)"), index (col) #2=2 ("索引 (列)"), index (col) #3=4 ("索引 (列)"), index (col) #4=5 ("索引 (列)")) -> (element #1=w462:string[], element #2=w460:string[], element #3=w448:string[], element #4=w447:string[])  [unwired: 4 in]
        n218 = for {
          tunnel: w462 -> [w504] mode=indexing
          tunnel: w444 -> [w503]
          shift-right: [w501] -> w457
          shift-left: w460 -> [w493]
          tunnel: w455 -> [w497]
          tunnel: [w496] -> w454
          shift-right: [w492] -> w445
          shift-left: w448 -> [w487]
          shift-right: [w491] -> w446
          shift-left: w447 -> [w489]
          i -> [w477]
          w472 = u32 3342591 ("颜色盒")
          w474 = T10 {"Row"=0, "Column"=0} ("活动单元格:活动单元格")
          n219 = case shown="\"灭火装置监测\"" w504 {
            tunnel: w503 -> [_ w525 w531 w537 w543 w549 w555 w561 w567 w572 w577 w583 w589]
            tunnel: [FALSE ("烟雾监测输出") w521 w527 w533 w539 w545 w551 w557 w563 w569 w574 w579 w585] -> w488
            tunnel: [_ w523 w529 w535 w541 w547 w553 w559 w565 w571 w576 w581 w587] -> w490
            tunnel: [FALSE ("crossing") w520 w526 w532 w538 w544 w550 w556 w562 w568 w573 w578 w584] -> w471
            frame "假", Default {
            }
            frame "市电监测" {
              n220 = Unbundle By Name(w525) -> ("自动重合闸输出"=w524:cluster{"自动重合闸告警":bool, "告警内容":string})
              n221 = Unbundle By Name(w524) -> ("自动重合闸告警"=w521:bool, "告警内容"=w523:string)
              n222 = call <vilib>:"Boolean Crossing PtByPt.vi"("direction"=enum16{"either", "false-true", "true-false"}."false-true", "input"=w521) -> ("crossing"=w520:bool)  [unwired: 1 in]
            }
            frame "空调监测" {
              n223 = Unbundle By Name(w531) -> ("空调监测输出"=w530:cluster{"空调监测告警":bool, "告警内容":string})
              n224 = Unbundle By Name(w530) -> ("空调监测告警"=w527:bool, "告警内容"=w529:string)
              n225 = call <vilib>:"Boolean Crossing PtByPt.vi"("direction"=enum16{"either", "false-true", "true-false"}."false-true", "input"=w527) -> ("crossing"=w526:bool)  [unwired: 1 in]
            }
            frame "漏水监测" {
              n226 = Unbundle By Name(w537) -> ("漏水监测输出"=w536:cluster{"漏水监测告警":bool, "告警内容":string})
              n227 = Unbundle By Name(w536) -> ("漏水监测告警"=w533:bool, "告警内容"=w535:string)
              n228 = call <vilib>:"Boolean Crossing PtByPt.vi"("direction"=enum16{"either", "false-true", "true-false"}."false-true", "input"=w533) -> ("crossing"=w532:bool)  [unwired: 1 in]
            }
            frame "门禁开关监测" {
              n229 = Unbundle By Name(w543) -> ("门禁监测输出"=w542:cluster{"门禁监测告警":bool, "告警内容":string})
              n230 = Unbundle By Name(w542) -> ("门禁监测告警"=w539:bool, "告警内容"=w541:string)
              n231 = call <vilib>:"Boolean Crossing PtByPt.vi"("direction"=enum16{"either", "false-true", "true-false"}."false-true", "input"=w539) -> ("crossing"=w538:bool)  [unwired: 1 in]
            }
            frame "温湿度监测" {
              n232 = Unbundle By Name(w549) -> ("温湿度监测输出"=w548:cluster{"温湿度监测告警":bool, "告警内容":string})
              n233 = Unbundle By Name(w548) -> ("温湿度监测告警"=w545:bool, "告警内容"=w547:string)
              n234 = call <vilib>:"Boolean Crossing PtByPt.vi"("direction"=enum16{"either", "false-true", "true-false"}."false-true", "input"=w545) -> ("crossing"=w544:bool)  [unwired: 1 in]
            }
            frame "烟雾监测" {
              n235 = Unbundle By Name(w555) -> ("烟雾监测输出"=w554:cluster{"烟雾监测告警":bool, "告警内容":string})
              n236 = Unbundle By Name(w554) -> ("烟雾监测告警"=w551:bool, "告警内容"=w553:string)
              n237 = call <vilib>:"Boolean Crossing PtByPt.vi"("direction"=enum16{"either", "false-true", "true-false"}."false-true", "input"=w551) -> ("crossing"=w550:bool)  [unwired: 1 in]
            }
            frame "UPS监测" {
              n238 = Unbundle By Name(w561) -> ("UPS输出"=w560:cluster{"UPS告警":bool, "告警内容":string})
              n239 = Unbundle By Name(w560) -> ("UPS告警"=w557:bool, "告警内容"=w559:string)
              n240 = call <vilib>:"Boolean Crossing PtByPt.vi"("direction"=enum16{"either", "false-true", "true-false"}."false-true", "input"=w557) -> ("crossing"=w556:bool)  [unwired: 1 in]
            }
            frame "蓄电池监测" {
              n241 = Unbundle By Name(w567) -> ("蓄电池输出"=w566:cluster{"蓄电池告警":bool, "告警内容":string})
              n242 = Unbundle By Name(w566) -> ("蓄电池告警"=w563:bool, "告警内容"=w565:string)
              n243 = call <vilib>:"Boolean Crossing PtByPt.vi"("direction"=enum16{"either", "false-true", "true-false"}."false-true", "input"=w563) -> ("crossing"=w562:bool)  [unwired: 1 in]
            }
            frame "GPS监测" {
              n244 = Unbundle By Name(w572) -> ("GPS输出.定位告警"=w569:bool, "GPS输出.告警内容"=w571:string)
              n245 = call <vilib>:"Boolean Crossing PtByPt.vi"("direction"=enum16{"either", "false-true", "true-false"}."false-true", "input"=w569) -> ("crossing"=w568:bool)  [unwired: 1 in]
            }
            frame "北斗监测" {
              n246 = Unbundle By Name(w577) -> ("北斗输出.定位告警"=w574:bool, "北斗输出.告警内容"=w576:string)
              n247 = call <vilib>:"Boolean Crossing PtByPt.vi"("direction"=enum16{"either", "false-true", "true-false"}."false-true", "input"=w574) -> ("crossing"=w573:bool)  [unwired: 1 in]
            }
            frame "气象监测" {
              n248 = Unbundle By Name(w583) -> ("气象输出"=w582:cluster{"气象告警":bool, "告警内容":string})
              n249 = Unbundle By Name(w582) -> ("气象告警"=w579:bool, "告警内容"=w581:string)
              n250 = call <vilib>:"Boolean Crossing PtByPt.vi"("direction"=enum16{"either", "false-true", "true-false"}."false-true", "input"=w579) -> ("crossing"=w578:bool)  [unwired: 1 in]
            }
            frame "灭火装置监测" {
              n251 = Unbundle By Name(w589) -> ("灭火装置输出"=w588:cluster{"灭火装置告警":bool, "告警内容":string})
              n252 = Unbundle By Name(w588) -> ("灭火装置告警"=w585:bool, "告警内容"=w587:string)
              n253 = call <vilib>:"Boolean Crossing PtByPt.vi"("direction"=enum16{"either", "false-true", "true-false"}."false-true", "input"=w585) -> ("crossing"=w584:bool)  [unwired: 1 in]
            }
          }
          n254 = Index Array(array=w487, index=w477) -> (element=w486:string)
          n255 = case shown="True" w488 {
            tunnel: ["正常" "报警"] -> w502
            tunnel: [u32 6618880 u32 16711680] -> w498
            tunnel: [u32 12369084 u32 3342591 ("颜色盒")] -> w480
            frame False {
            }
            frame True {
            }
          }
          n256 = case shown="False" w471 {
            tunnel: [w505 w506] -> w485
            tunnel: w486 -> [w505 _]
            frame False {
            }
            frame True {
              n257 = Get Date/Time In Seconds() -> (seconds since 1Jan1904=w511:timestamp)
              n258 = Get Date/Time String(date format (0)=enum16{"short", "long", "abbreviated"}."long" ("日期格式(0)"), seconds (now)=w511, want seconds? (F)=TRUE ("需要秒？(F)")) -> (date string=w508:string, time string=w507:string)
              n259 = Concatenate Strings(w508, w507) -> (w506:string)
            }
          }
          n260 = Replace Array Subset(array=w489, new element=w490, index=w477) -> (w491:string[])
          n261 = Bundle By Name(cluster=w474, "Row"=w477, "Column"=2) -> (w499:T10)
          n262 = Bundle By Name(cluster=w474, "Row"=w477, "Column"=6) -> (w494:T10)
          n263 = Bundle By Name(cluster=w474, "Row"=w477, "Column"=4) -> (w482:T10)
          n264 = Bundle By Name(cluster=w474, "Row"=w477, "Column"=5) -> (w481:T10)
          n265 = Bundle By Name(cluster=w474, "Row"=w477, "Column"=1) -> (w476:T10)
          n266 = Bundle By Name(cluster=w474, "Row"=w477, "Column"=3) -> (w473:T10)
          n267 = Replace Array Subset(array=w493, new element=w502, index=w477) -> (w501:string[])
          n268 = property on="设备列表" class="MCListbox (strict)"(error in=w497, "ActiveCell"=w499, "CellFontColor"=w498, "ActiveCell"=w494, "CellFontColor"=w480, "ActiveCell"=w482, "CellFontColor"=w480, "ActiveCell"=w481, "CellFontColor"=w480, "ActiveCell"=w476, "CellFontBold"=TRUE ("活动单元格:单元格字体:粗体"), "CellFontColor"=w472, "ActiveCell"=w473, "CellFontColor"=w472) -> (error out=w496:errorcluster)  [unwired: 1 in, 1 out]
          n269 = Replace Array Subset(array=w487, new element=w485, index=w477) -> (w492:string[])
        }
        n270 = Index Array(array=w470) -> (element=w465:i32)  [unwired: 1 in]
        "当前传感器数量:" <- w465
        n271 = for {
          N: w465 -> [_]
          tunnel: [w590] -> w469 mode=indexing
          i -> [w591]
          n272 = Increment(x=w591) -> (x+1=w590:i32)
        }
        n273 = Number To Decimal String(number=w469) -> (decimal integer string=w468:string[])  [unwired: 1 in]
        n274 = Replace Array Subset(array=w464, new element=w468, index (col)=0 ("禁用的索引 (列)")) -> (w459:string[][])  [unwired: 1 in]
        n275 = Replace Array Subset(array=w459, new element #1=w457, index (col) #1=2 ("禁用的索引 (列)"), new element #2=w445, index (col) #2=4 ("索引 (列)"), new element #3=w446, index (col) #3=5 ("索引 (列)")) -> (w456:string[][])  [unwired: 3 in]
        n276 = property on="设备列表" class="MCListbox (strict)"(error in=w454, "ItemNames"=w456) -> ()  [unwired: 1 in, 2 out]
      }
      event "add": Value Change {
        w594 = u32 3342591 ("颜色盒")
        n277 = event-data() -> ()  [unwired: 1 in, 6 out]
        n278 = property class="MCListbox (strict)"(reference=w618) -> (reference out=w607:refnum<vi>, "ItemNames"=w611:string[][])  [unwired: 1 in, 1 out]
        n279 = property class="Enum (strict)"(reference=w617) -> ("RingText.Text"=w616:string)  [unwired: 1 in, 2 out]
        n280 = Array Size(array=w611) -> (size(s)=w610:i32[])
        n281 = Index Array(array=w610) -> (element=w599:i32)  [unwired: 1 in]
        n282 = Increment(x=w599) -> (x+1=w609:i32)
        n283 = Number To Decimal String(number=w609) -> (decimal integer string=w608:string)  [unwired: 1 in]
        n284 = Build Array(w608, w616, "正常" ("元素"), "点击查看详情" ("元素"), "解除告警" ("元素")) -> (w615:string[])
        n285 = Build Array (concatenate)(w611, w615) -> (w596:string[][])
        n286 = Bundle(w599, "Column"=1) -> (w595:cluster{i32, "Column":i32})  [unwired: 1 in]
        n287 = Bundle(w599, "Column"=2) -> (w604:cluster{i32, "Column":i32})  [unwired: 1 in]
        n288 = Bundle(w599, "Column"=3) -> (w601:cluster{i32, "Column":i32})  [unwired: 1 in]
        n289 = Bundle(w599, "Column"=4) -> (w598:cluster{i32, "Column":i32})  [unwired: 1 in]
        n290 = property class="MCListbox (strict)"(reference=w607, "ItemNames"=w596, "ActiveCell"=w595, "CellFontColor"=w594, "CellFontBold"=TRUE ("活动单元格:单元格字体:斜体"), "ActiveCell"=w604, "CellFontColor"=u32 61277 ("颜色盒"), "ActiveCell"=w601, "CellFontColor"=w594, "ActiveCell"=w598, "CellFontColor"=u32 12369084 ("颜色盒")) -> ()  [unwired: 1 in, 2 out]
      }
      event "设备列表": Mouse Down {
        n291 = event-data() -> ("CtlRef"=w631:refnum<vi>, "Coords"=w629:T11)  [unwired: 1 in, 6 out]
        n292 = property class="MCListbox (strict)"(reference=w625) -> (reference out=w621:refnum<vi>, "ItemNames"=w624:string[][])  [unwired: 1 in, 1 out]
        n293 = invoke class="MCListbox (strict)" method="Point To Row Column"(reference=w631, "Point"=w629) -> ("CellPosition"=w628:T10)  [unwired: 5 in, 6 out]
        n294 = Unbundle By Name(w628) -> ("Row"=w627:i32, "Column"=w630:i32)
        n295 = Array Size(array=w624) -> (size(s)=w623:i32[])
        n296 = Index Array(array=w623) -> (element=w622:i32)  [unwired: 1 in]
        n297 = In Range and Coerce(upper limit=w622, x=w627, lower limit=0 ("下限")) -> (In Range?=w620:bool)  [unwired: 1 out]
        n298 = case shown="True" w620 {
          tunnel: w630 -> [_ w641]
          tunnel: w627 -> [_ w640]
          tunnel: w628 -> [_ w638]
          tunnel: w621 -> [_ w635]
          tunnel: w619 -> [_ w632]
          frame False {
          }
          frame True {
            # "非列首字符串"
            n299 = property class="MCListbox (strict)"(reference=w635, "CellBG"=u32 16777216) -> (reference out=w636:refnum<vi>)  [unwired: 1 in, 1 out]
            n300 = property class="MCListbox (strict)"(reference=w636, "ActiveCell"=w638, "CellBG"=u32 16777216) -> (reference out=w639:refnum<vi>, "ItemNames"=w642:string[][], "CellFontColor"=w633:u32)  [unwired: 1 in, 1 out]
            n301 = case shown="6" w641 {
              tunnel: w642 -> [_ w650 w715]
              tunnel: w640 -> [_ w648 w713]
              tunnel: w639 -> [_ _ w714]
              tunnel: w633 -> [_ _ w712]
              tunnel: w632 -> [_ w646 _]
              frame 0, Default {
              }
              frame 3 {
                # "查看详情分支"
                n302 = Index Array(array=w650, index (row)=w648, index (col)=1 ("禁用的索引 (列)")) -> (element=w647:string)
                n303 = case shown="\"市电监测\"" w647 {
                  selector: w647 -> [w651 _ _ _ _ _ _ _ _ _ _ _ _ _ _ _ _ _ _ _]
                  tunnel: w646 -> [_ w655 w658 w661 w664 w667 w670 w673 w676 w679 w681 w684 w687 w690 w693 w696 w699 w702 w705 w708]
                  tunnel: [_ w654 w656 w659 w662 w665 w668 w671 w674 w677 w680 w683 w686 w689 w692 w695 w698 w701 w704 w707] -> w643
                  frame "假", Default {
                    n304 = Concatenate Strings(w651, "详情" ("字符串")) -> (w653:string)
                    n305 = One Button Dialog(message=w653) -> ()  [unwired: 1 in, 1 out]
                  }
                  frame "市电监测" {
                    n306 = Index Array(array=w655) -> (element=w654:refnum<vi>)  [unwired: 1 in]
                  }
                  frame "用水量监测" {
                    n307 = Index Array(array=w658, index=1 ("索引")) -> (element=w656:refnum<vi>)
                  }
                  frame "烟雾监测" {
                    (unwired) T9."Standard" ("状态")
                    n308 = Index Array(array=w661, index=2 ("索引")) -> (element=w659:refnum<vi>)
                  }
                  frame "温湿度监测" {
                    (unwired) T9."Standard" ("状态")
                    n309 = Index Array(array=w664, index=3 ("索引")) -> (element=w662:refnum<vi>)
                  }
                  frame "振动监测" {
                    (unwired) T9."Standard" ("状态")
                    n310 = Index Array(array=w667, index=4 ("索引")) -> (element=w665:refnum<vi>)
                  }
                  frame "红外入侵监测" {
                    (unwired) T9."Standard" ("状态")
                    n311 = Index Array(array=w670, index=5 ("索引")) -> (element=w668:refnum<vi>)
                  }
                  frame "漏水监测" {
                    (unwired) T9."Standard" ("状态")
                    n312 = Index Array(array=w673, index=6 ("索引")) -> (element=w671:refnum<vi>)
                  }
                  frame "门禁开关监测" {
                    (unwired) T9."Standard" ("状态")
                    n313 = Index Array(array=w676, index=7 ("索引")) -> (element=w674:refnum<vi>)
                  }
                  frame "门禁开关监测2" {
                    (unwired) T9."Standard" ("状态")
                    n314 = Index Array(array=w679, index=8 ("索引")) -> (element=w677:refnum<vi>)
                  }
                  frame "视频监测" {
                    (unwired) T9."Standard" ("状态")
                    n315 = Index Array(array=w681, index=9 ("索引")) -> (element=w680:refnum<vi>)
                  }
                  frame "UPS监测" {
                    (unwired) T9."Standard" ("状态")
                    n316 = Index Array(array=w684, index=10 ("索引")) -> (element=w683:refnum<vi>)
                  }
                  frame "空调监测" {
                    (unwired) T9."Standard" ("状态")
                    n317 = Index Array(array=w687, index=11 ("索引")) -> (element=w686:refnum<vi>)
                  }
                  frame "冰箱监测" {
                    (unwired) T9."Standard" ("状态")
                    n318 = Index Array(array=w690, index=12 ("索引")) -> (element=w689:refnum<vi>)
                  }
                  frame "排气扇监测" {
                    (unwired) T9."Standard" ("状态")
                    n319 = Index Array(array=w693, index=13 ("索引")) -> (element=w692:refnum<vi>)
                  }
                  frame "蓄电池监测" {
                    (unwired) T9."Standard" ("状态")
                    n320 = Index Array(array=w696, index=14 ("索引")) -> (element=w695:refnum<vi>)
                  }
                  frame "蓄电池监测2" {
                    (unwired) T9."Standard" ("状态")
                    n321 = Index Array(array=w699, index=15 ("索引")) -> (element=w698:refnum<vi>)
                  }
                  frame "GPS监测" {
                    (unwired) T9."Standard" ("状态")
                    n322 = Index Array(array=w702, index=16 ("索引")) -> (element=w701:refnum<vi>)
                  }
                  frame "北斗监测" {
                    (unwired) T9."Standard" ("状态")
                    n323 = Index Array(array=w705, index=17 ("索引")) -> (element=w704:refnum<vi>)
                  }
                  frame "气象监测" {
                    (unwired) T9."Standard" ("状态")
                    n324 = Index Array(array=w708, index=18 ("索引")) -> (element=w707:refnum<vi>)
                  }
                }
                n325 = invoke class="VI" method="FP.Open"(reference=w643, "Activate"=TRUE ("激活？"), "State"=T9."Standard" ("状态")) -> ()  [unwired: 2 in, 5 out]
              }
              frame 6 {
                # "解除报警"
                n326 = Equal?(x=w712, y=u32 3342591 ("颜色盒")) -> (x = y?=w711:bool)
                n327 = case shown="True" w711 {
                  tunnel: w715 -> [_ w720]
                  tunnel: w714 -> [_ _]
                  tunnel: w713 -> [_ w719]
                  frame False {
                  }
                  frame True {
                    n328 = Index Array(array=w720, index (row)=w719, index (col)=1 ("禁用的索引 (列)")) -> (element=w716:string)
                    n329 = Format Into String(format string="是否解除%s报警？" ("消息"), w716) -> (resulting string=w721:string)  [unwired: 2 in, 1 out]
                    n330 = Two Button Dialog(message=w721) -> (T button?=w717:bool)  [unwired: 2 in]
                    n331 = case shown="True" w717 {
                      tunnel: w716 -> [_ w725]
                      frame False {
                      }
                      frame True {
                        # "触发解除报警事件"
                        n332 = global read "内部交互全局变量.vi" "监测配置输出"() -> (w724:T3)
                        n333 = case shown="\"灭火装置监测\"" w725 {
                          tunnel: w724 -> [w727 w730 w733 w736 w739 w741 w745 w748 w750 w753 w756 w759 w762 w765]
                          tunnel: [w727 w729 w732 w735 w738 w740 w743 w747 w749 w752 w755 w758 w761 w764] -> w723
                          tunnel: FALSE ("烟雾监测输出") -> [_ w728 w731 w734 w737 w742 w744 w746 w751 w754 w757 w760 w763 w766]
                          frame "假", Default {
                          }
                          frame "市电监测" {
                            n334 = Bundle By Name(cluster=w730, "自动重合闸输出.自动重合闸告警"=w728) -> (w729:T3)
                          }
                          frame "空调监测" {
                            n335 = Bundle By Name(cluster=w733, "空调监测输出.空调监测告警"=w731) -> (w732:T3)
                          }
                          frame "漏水监测" {
                            n336 = Bundle By Name(cluster=w736, "漏水监测输出.漏水监测告警"=w734) -> (w735:T3)
                          }
                          frame "门禁开关监测" {
                            n337 = Bundle By Name(cluster=w739, "门禁监测输出.门禁监测告警"=w737) -> (w738:T3)
                          }
                          frame "温湿度监测" {
                            n338 = Bundle By Name(cluster=w741, "温湿度监测输出.温湿度监测告警"=w742) -> (w740:T3)
                          }
                          frame "烟雾监测" {
                            n339 = Bundle By Name(cluster=w745, "烟雾监测输出.烟雾监测告警"=w744) -> (w743:T3)
                          }
                          frame "UPS监测" {
                            n340 = Bundle By Name(cluster=w748, "UPS输出.UPS告警"=w746) -> (w747:T3)
                          }
                          frame "蓄电池监测" {
                            n341 = Bundle By Name(cluster=w750, "蓄电池输出.蓄电池告警"=w751) -> (w749:T3)
                          }
                          frame "蓄电池监测2" {
                            n342 = Bundle By Name(cluster=w753, "蓄电池输出2.蓄电池告警"=w754) -> (w752:T3)
                          }
                          frame "GPS监测" {
                            n343 = Bundle By Name(cluster=w756, "GPS输出.定位告警"=w757) -> (w755:T3)
                          }
                          frame "北斗监测" {
                            n344 = Bundle By Name(cluster=w759, "北斗输出.定位告警"=w760) -> (w758:T3)
                          }
                          frame "气象监测" {
                            n345 = Bundle By Name(cluster=w762, "气象输出.气象告警"=w763) -> (w761:T3)
                          }
                          frame "灭火装置监测" {
                            n346 = Bundle By Name(cluster=w765, "灭火装置输出.灭火装置告警"=w766) -> (w764:T3)
                          }
                        }
                        n347 = global write "内部交互全局变量.vi" "监测配置输出"(w723) -> ()
                      }
                    }
                  }
                }
              }
            }
          }
        }
      }
      event "监测设备更新": Value Change {
        n348 = event-data() -> ()  [unwired: 1 in, 6 out]
        n349 = global read "断电保存全局变量.vi" "监测设备配置"() -> (w770:T2)
        n350 = Cluster To Array(cluster=w770) -> (array=w773:bool[])
        n351 = for {
          tunnel: w772 -> [w776] mode=indexing
          tunnel: [w775] -> w771 mode=indexing
          tunnel: w773 -> [w777] mode=indexing
          tunnel: [w774] -> w769
          n352 = case shown="True" w777 {
            tunnel: w776 -> [w780 w783]
            tunnel: [w779 w785] -> w775
            tunnel: [w778 w784] -> w774
            frame False {
              n353 = invoke class="VI" method="Abort VI"(reference=w780) -> (reference out=w779:refnum<vi>, error out=w778:errorcluster)  [unwired: 2 in, 1 out]
            }
            frame True {
              n354 = property class="VI"(reference=w783) -> (reference out=w781:refnum<vi>, "Exec.State"=w782:T12)  [unwired: 1 in, 1 out]
              n355 = case shown="\"Idle\"" w782 {
                tunnel: [w786 w789] -> w785
                tunnel: [_ w788] -> w784
                tunnel: w781 -> [w786 w787]
                frame "Bad", Default {
                }
                frame "Idle" {
                  n356 = invoke class="VI" method="Run VI"(reference=w787, "Wait until done"=FALSE ("结束前等待"), "Auto Dispose Ref"=FALSE ("自动销毁引用")) -> (reference out=w789:refnum<vi>, error out=w788:errorcluster)  [unwired: 2 in, 3 out]
                }
              }
            }
          }
        }
        n357 = call <vilib>:"Clear Errors.vi"("error in (no error)"=w769) -> ("error out"=w768:errorcluster)  [unwired: 5 in, 1 out]
        n358 = call "save.vi"("error in (no error)"=w768) -> ("error out"=w767:errorcluster)  [unwired: 10 in]
      }
    }
  }
